vi "ukol 3.vi"() -> ()   [LabVIEW 2023]
uses:
  <vilib>/Analysis/2dsp.llb/1D Cross Correlation (DBL).vi
  <vilib>/Analysis/NI_AALPro.lvlib
panel:
  out "max index(es) 2":i32
  out "max index(es)":i32
  out "x-y 3":i32
  out "Waveform Graph 6":dbl[][](graph)
  out "x-y 2":i32
  out "Waveform Graph 5":dbl[][](graph)
  out "Waveform Graph 4":dbl[](graph)
  out "Waveform Graph 3":dbl[](graph)
  out "Waveform Graph 2":waveform(dbl)(graph)
  out "Waveform Graph":waveform(dbl)(graph)
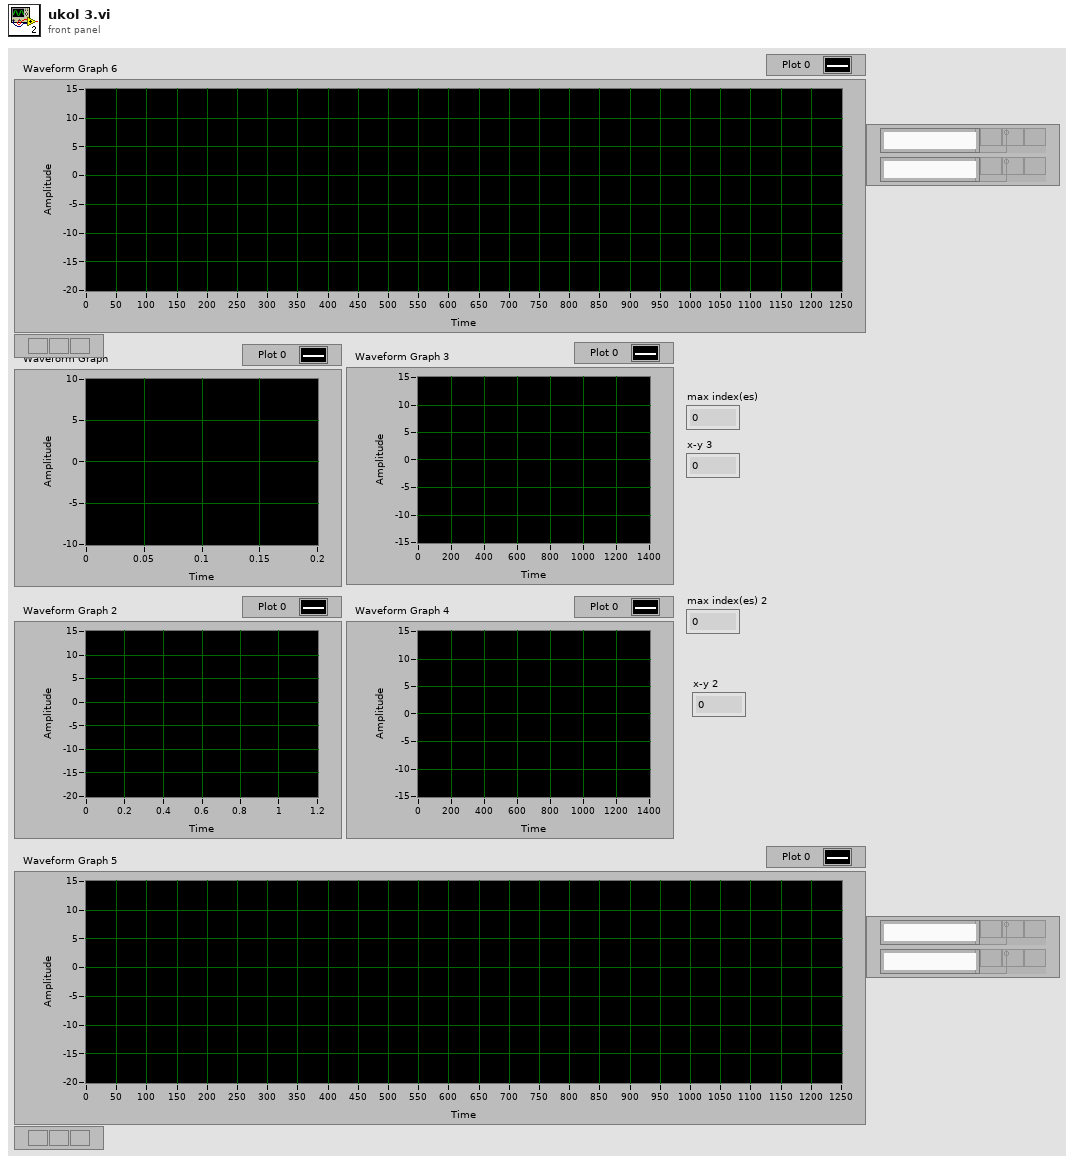
[diagram p1: front panel]
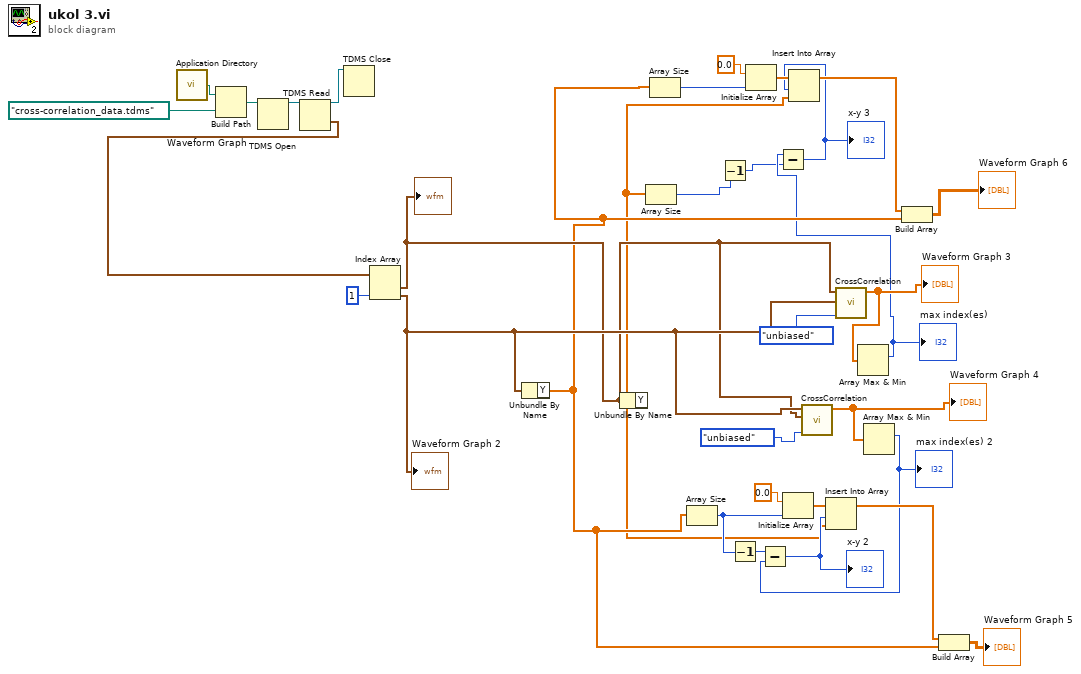
[diagram p0: block diagram]
diagram:
  n1 = call <vilib>:"Application Directory.vi"() -> ("Application Directory"=w32:path)
  n2 = Build Path(base path=w32, name or relative path=path "cross-correlation_data.tdms") -> (appended path=w27:path)
  n3 = TDMS Open(11:w27) -> (3:w30:refnum<k34>)  [unwired: 6 in, 1 out]
  n4 = TDMS Read(0:w30) -> (4:w29:refnum<k34>, 10:w28:waveform(dbl)[])  [unwired: 7 in, 4 out]
  n5 = TDMS Close(11:w29) -> ()  [unwired: 1 in, 2 out]
  n6 = Index Array(array=w28, index #2=1 ("index")) -> (element #1=w19:waveform(dbl), element #2=w20:waveform(dbl))  [unwired: 1 in]
  "Waveform Graph" <- w19
  "Waveform Graph 2" <- w20
  n7 = Unbundle By Name(w20) -> ("Y"=w7:dbl[])
  n8 = Unbundle By Name(w19) -> ("Y"=w6:dbl[])
  n9 = Array Size(array=w6) -> (size(s)=w3:i32)
  n10 = Array Size(array=w7) -> (size(s)=w5:i32)
  n11 = Array Size(array=w7) -> (size(s)=w16:i32)
  n12 = Decrement(x=w3) -> (x-1=w2:i32)
  n13 = Decrement(x=w16) -> (x-1=w15:i32)
  n14 = Initialize Array(0.0 ("element"), w5) -> (w9:dbl[])
  n15 = Initialize Array(0.0 ("element"), w16) -> (w17:dbl[])
  n16 = call-poly <vilib>:"CrossCorrelation.vi"("normalization"=enum32{"none", "unbiased", "biased"}."unbiased", "Y"=w19, "X"=w20) -> ("Rxy"=w22:dbl[])  [unwired: 7 in, 1 out]
  "Waveform Graph 4" <- w22
  n17 = call-poly <vilib>:"CrossCorrelation.vi"("normalization"=enum32{"none", "unbiased", "biased"}."unbiased", "Y"=w20, "X"=w19) -> ("Rxy"=w23:dbl[])  [unwired: 7 in, 1 out]
  "Waveform Graph 3" <- w23
  n18 = Array Max & Min(array=w23) -> (max index (indices)=w4:i32)  [unwired: 3 out]
  "max index(es)" <- w4
  n19 = Subtract(x=w4, y=w2) -> (x-y=w1:i32)
  "x-y 3" <- w1
  n20 = Insert Into Array(array=w9, index=w1, new element=w6) -> (w8:dbl[])
  n21 = Array Max & Min(array=w22) -> (max index (indices)=w12:i32)  [unwired: 3 out]
  "max index(es) 2" <- w12
  n22 = Subtract(x=w15, y=w12) -> (x-y=w14:i32)
  "x-y 2" <- w14
  n23 = Insert Into Array(array=w17, index=w14, new element=w6) -> (w13:dbl[])
  n24 = Build Array(w8, w7) -> (→"Waveform Graph 6":dbl[][])
  n25 = Build Array(w13, w7) -> (→"Waveform Graph 5":dbl[][])
